vi "host_scan_counter.vi"(7 "reset?":bool, 10 "update?":bool, 11 "count up?":bool) -> (3 "finished?":bool)   [LabVIEW 2021]
panel:
  out "counter":i32
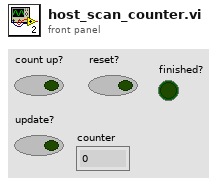
[diagram p1: front panel]
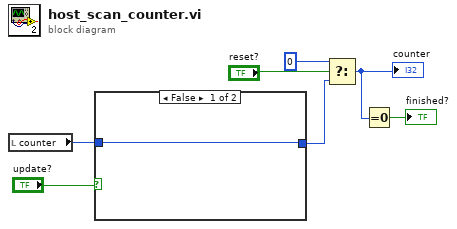
[diagram p0: block diagram]
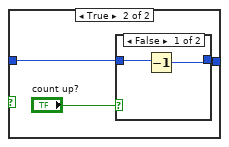
[diagram p2: hidden frame]
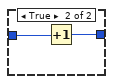
[diagram p3: hidden frame]
diagram:
  n1 = local read "counter"() -> (w6:i32)
  n2 = case shown="False" "update?" {
    tunnel: w6 -> [w8 w10]
    tunnel: [w8 w9] -> w5
    frame False {
    }
    frame True {
      n3 = case shown="False" "count up?" {
        tunnel: w10 -> [w13 w15]
        tunnel: [w12 w14] -> w9
        frame False {
          n4 = Decrement(x=w13) -> (x-1=w12:i32)
        }
        frame True {
          n5 = Increment(x=w15) -> (x+1=w14:i32)
        }
      }
    }
  }
  n6 = Select(t=0, s="reset?", f=w5) -> (s? t:f=w3:i32)
  "counter" <- w3
  n7 = Equal To 0?(x=w3) -> (x = 0?=→"finished?":bool)
